vi "Incoming Signals.vi"(8 "error in (no error)":errorcluster, 11 "Node Ptr":T3 format="%.0x") -> (0 "error out":errorcluster)   [LabVIEW 2009, in "NI-XNET Custom Device.lvlib"]
uses:
  NI-XNET Custom Device.lvlib
  <vilib>/NI VeriStand/Custom Device API/Custom Device Item Ref.ctl
  Add Selected.ctl
  Add All.ctl
  <vilib>/NI VeriStand/Custom Device API/Custom Device Channel.ctl
  <vilib>/NI VeriStand/Custom Device API/Custom Device Channel Type.ctl
  <vilib>/NI VeriStand/Custom Device API/Set Item Property (Variant).vi
  <vilib>/xnet/xnet.llb/XNET String To IO Name (Frame).vi
  <vilib>/NI VeriStand/Custom Device API/Get Item Property (String).vi
  <vilib>/NI VeriStand/Custom Device API/Custom Device API.lvlib
  Program Files/National Instruments/LabVIEW 2009/resource/objmgr/xnet.rc
panel:
  in  "Add All":T1
  in  "Add Signal":T2
  in  "Header 4":cluster{"Section Name":string}={"Section Name"="Signal Specifications"}
  in  "Header 3":cluster{"Section Name":string}={"Section Name"="Signal Values"}
  in  "Header 2":cluster{"Section Name":string}={"Section Name"="Signal Settings"}
  out "Unit":string
  out "Start Bit":u32
  out "Scaling Offset":dbl
  out "Scaling Factor":dbl
  out "Number of Bits":u32
  out "Minimum Value":dbl
  out "Maximum Value":dbl
  out "Default Value":dbl
  out "Data Type":u32(ring) items=["Signed", "Unsigned", "IEEE Float"]
  out "Comment":string
  out "Byte Order":u32(ring) items=["Little Endian", "Big Endian"]
  in  "Signal Selection":i32(listbox)
  in  "Header":cluster{"Section Name":string}={"Section Name"="Signal Selection"}
  in  "Delete":bool
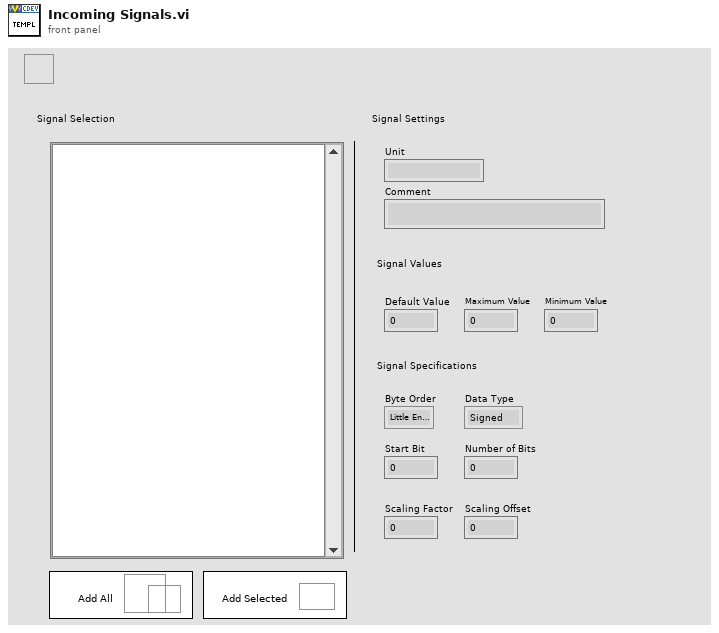
[diagram p1: front panel]
types:
  T1 = typedef "NI-XNET Custom Device.lvlib/Add All.ctl" = bool
  T2 = typedef "NI-XNET Custom Device.lvlib/Add Selected.ctl" = bool
  T3 = typedef "Custom Device API.lvlib/Custom Device Item Ref.ctl" = u64
  T4 = typedef "Custom Device API.lvlib/Custom Device Channel.ctl" = cluster{"Type":T5, "Units":string, "Default Value":dbl, "Faultable":bool, "Scalable":bool}
  T5 = typedef "Custom Device API.lvlib/Custom Device Channel Type.ctl" = enum16{"Input", "Output"}
  T6 = typedef "Custom Device API.lvlib/Custom Device Commands.ctl" = enum16{"Default", "Item renamed", "Shutdown"}
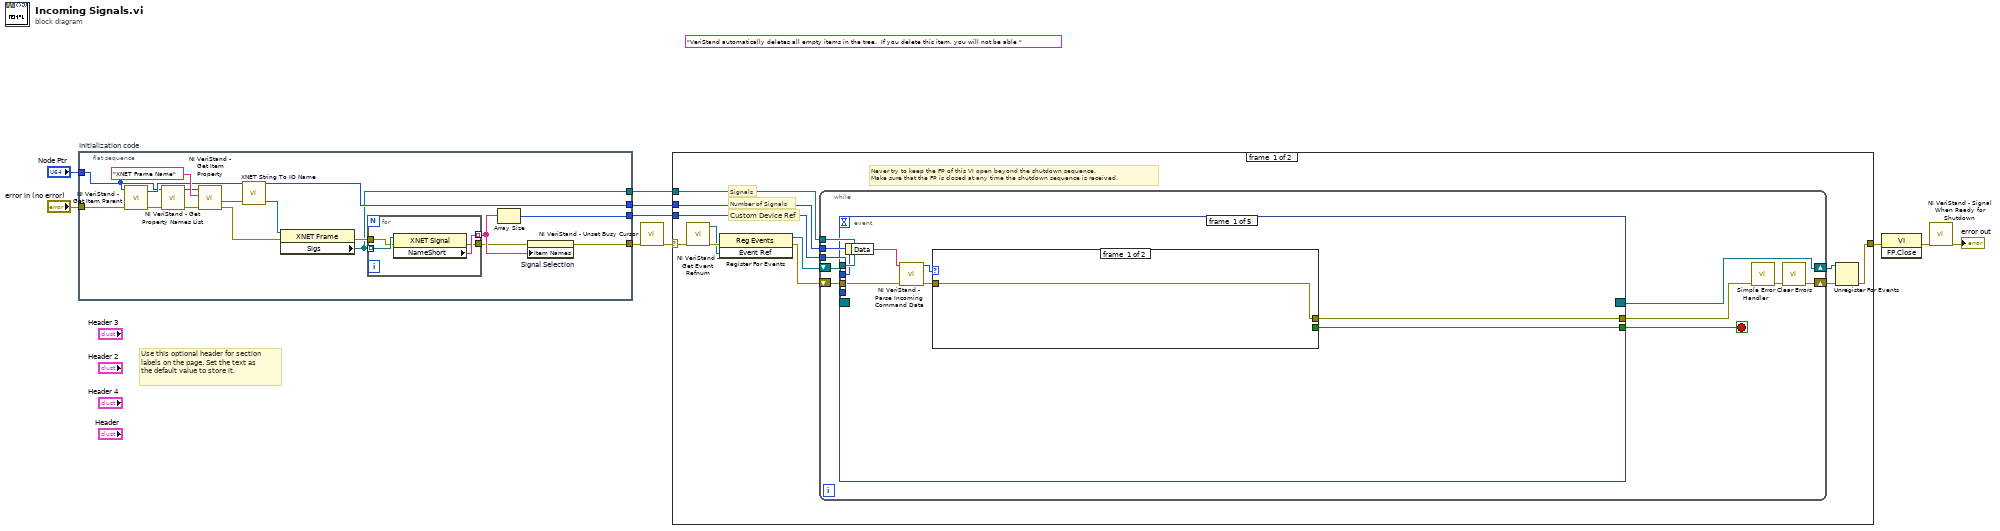
[diagram p0: block diagram]
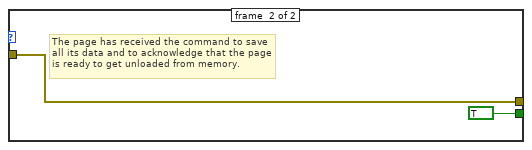
[diagram p2: hidden frame]
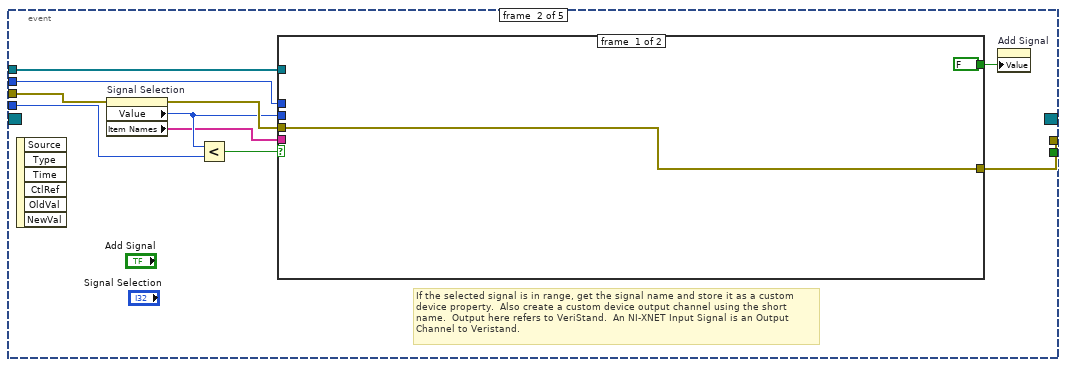
[diagram p3: hidden frame]
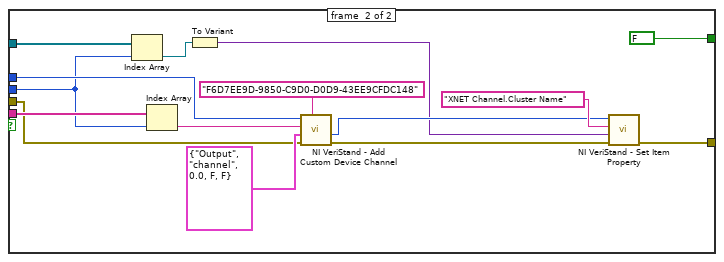
[diagram p4: hidden frame]
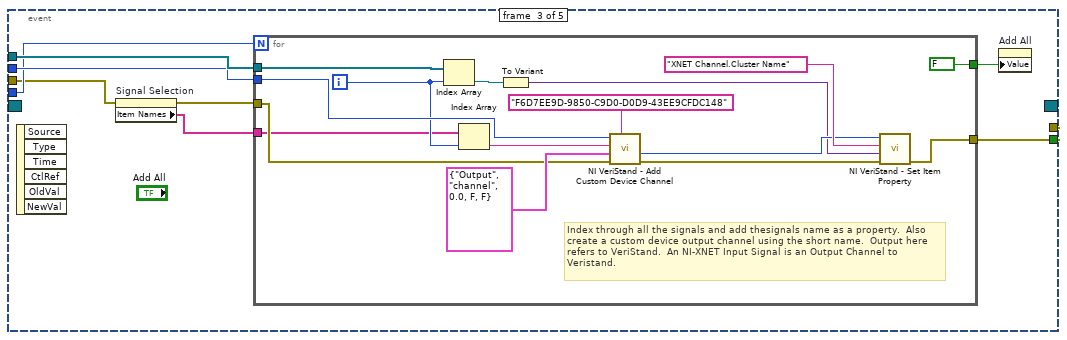
[diagram p5: hidden frame]
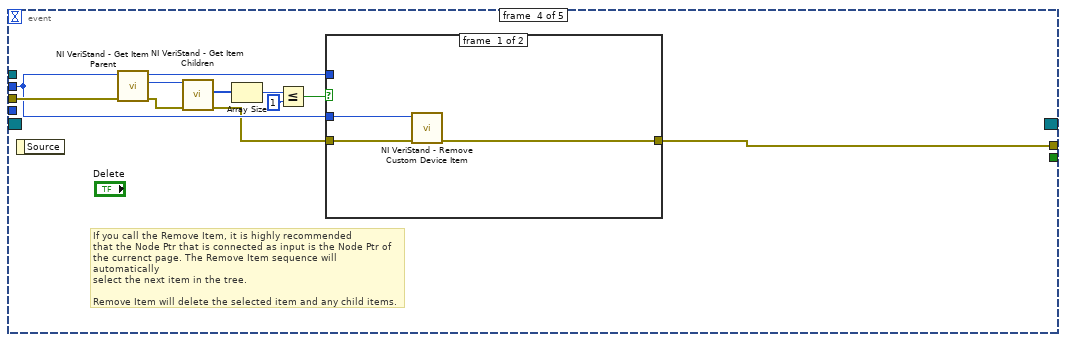
[diagram p6: hidden frame]
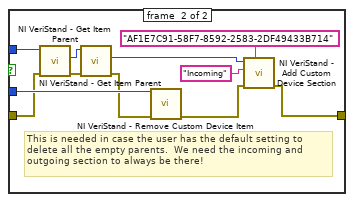
[diagram p7: hidden frame]
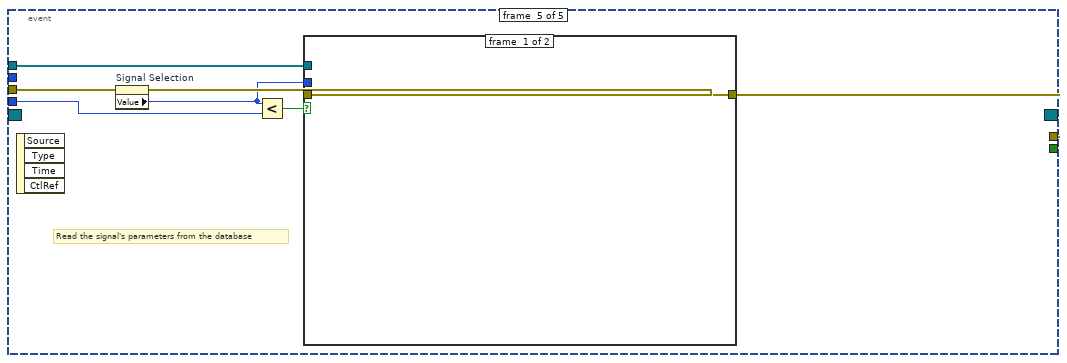
[diagram p8: hidden frame]
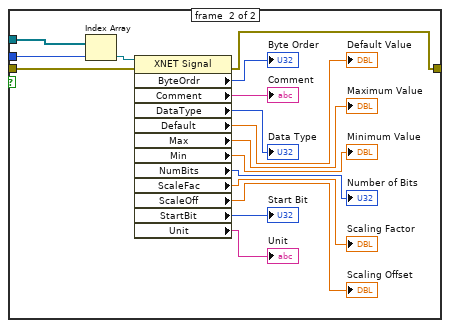
[diagram p9: hidden frame]
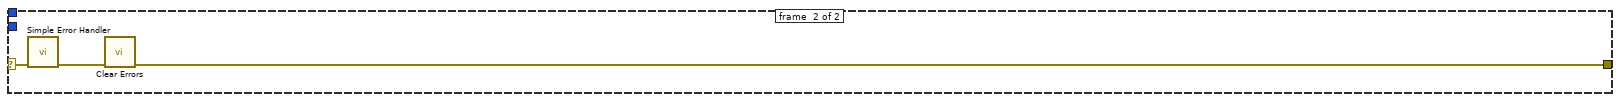
[diagram p10: hidden frame]
diagram:
  (unwired) "VeriStand automatically deletes all empty items in the tree.  If you delete this item, you will not be able " ("message")
  # "Use this optional header for section labels on the page. Set the text as the default value to store it."
  n1 = flat-sequence "Initialization code" {
    tunnel: "error in (no error)" -> [w14]
    tunnel: "Node Ptr" -> [w15]
    tunnel: [w18] -> w4
    tunnel: [w17] -> w3
    tunnel: [w16] -> w2
    tunnel: [w12] -> w1
    frame #0 {
      n2 = call <vilib>:"NI VeriStand - Get Item Parent.vi"("error in (no error)"=w14, "Parent Ref in"=w15) -> ("error out"=w25:errorcluster, "Parent Ref out"=w18:T3)  [unwired: 6 in, 2 out]
      n3 = call <vilib>:"NI VeriStand - Get Property Names List.vi"("error in (no error)"=w25, "Item Ref in"=w15) -> ("error out"=w23:errorcluster, "Item Ref out"=w24:T3)  [unwired: 7 in, 1 out]
      n4 = call-poly <vilib>:"NI VeriStand - Get Item Property.vi"("error in (no error)"=w23, "Property Name"="XNET Frame Name", "Item Ref in"=w24) -> ("error out"=w21:errorcluster, "Value"=w19:string)  [unwired: 5 in, 2 out]
      n5 = call-poly <vilib>:"XNET String To IO Name.vi"("string"=w19) -> ("XNET Frame"=w22:refnum<k21>)  [unwired: 4 in]
      n6 = property class="XNET Frame"(reference=w22, error in=w21) -> (error out=w20:errorcluster, "Sigs"=w17:refnum<k21>[])  [unwired: 1 out]
      n7 = for {
        tunnel: w17 -> [w30] mode=indexing
        tunnel: [w29] -> w13 mode=indexing
        tunnel: w20 -> [w28]
        tunnel: [w27] -> w11
        n8 = property class="XNET Signal"(reference=w30, error in=w28) -> (error out=w27:errorcluster, "NameShort"=w29:string)  [unwired: 1 out]
      }
      n9 = Array Size(array=w13) -> (size(s)=w16:i32)
      n10 = property on="Signal Selection" class="LstBox (strict)"(error in=w11, "Item Names"=w13) -> (error out=w12:errorcluster)  [unwired: 1 in, 1 out]
    }
  }
  n11 = call <vilib>:"NI VeriStand - Unset Busy Cursor.vi"("error in (no error)"=w1) -> ("error out"=w6:errorcluster)  [unwired: 10 out]
  n12 = case shown="No Error" w6 {
    selector: w6 -> [w34 w162]
    tunnel: [w38 w160] -> w10
    tunnel: w4 -> [w32 _]
    tunnel: w3 -> [w33 _]
    tunnel: w2 -> [w31 _]
    frame #0 {
      # "Custom Device Ref"
      # "Number of Signals"
      # "Signals"
      # "Never try to keep the FP of this VI open beyond the shutdown sequence.\nMake sure that the FP is closed at any time the shutdown sequence is received."
      n13 = call <vilib>:"NI VeriStand - Get Event Refnum.vi"("error in (no error)"=w34) -> ("error out"=w41:errorcluster, "Event Ref"=w37:refnum<user-event>)  [unwired: 9 out]
      n14 = register-events(error in=w41, w37) -> (reference out=w35:refnum<event-registration>, error out=w36:errorcluster)  [unwired: 1 in]
      n15 = while {
        shift-right: [w45] -> w39
        shift-left: w36 -> [w50]
        shift-right: [w51] -> w40
        shift-left: w35 -> [w49]
        tunnel: w33 -> [w44]
        tunnel: w32 -> [w43]
        tunnel: w31 -> [w42]
        stop <- w48 stop-if-true
        n16 = event shown="[3] \"Delete\": Value Change" {
          selector: w49 -> [_ _ _ _ _]
          dyn-events: [_ _ _ _ _] -> w51
          timeout: _ -> [_ _ _ _ _]
          tunnel: w50 -> [w57 w68 w89 w120 w140]
          tunnel: [w53 _ _ _ _] -> w48
          tunnel: [w52 w67 w93 w121 w141] -> w47
          tunnel: w44 -> [_ w70 w95 _ w142]
          tunnel: w43 -> [_ w69 w94 w119 _]
          tunnel: w42 -> [_ w65 w92 _ w138]
          event #0 {
            n17 = event-data() -> ("Data"=w56:string)  [unwired: 1 out]
            n18 = call <vilib>:"NI VeriStand - Parse Incoming Command Data.vi"("error in (no error)"=w57, "Data"=w56) -> ("error out"=w55:errorcluster, "Action"=w54:T6)  [unwired: 8 out]
            n19 = case shown="\"Shutdown\"" w54 {
              tunnel: w55 -> [w58 w59]
              tunnel: [_ TRUE] -> w53
              tunnel: [w58 w59] -> w52
              frame #0 {
              }
              frame #1 {
                # "The page has received the command to save all its data and to acknowledge that the page is ready to get unloaded from memory."
              }
            }
          }
          event #1 {
            # "If the selected signal is in range, get the signal name and store it as a custom device property.  Also create a custom device output channel using the short name.  Output here refers to VeriStand.  An NI-XNET Input Signal is an Output Channel to Veristand."
            n20 = event-data() -> ()  [unwired: 7 out]
            n21 = property on="Signal Selection" class="LstBox (strict)"(error in=w68) -> (error out=w66:errorcluster, "Value"=w62:i32, "Item Names"=w61:string[])  [unwired: 1 in, 1 out]
            n22 = Less?(x=w62, y=w65) -> (x < y?=w64:bool)
            n23 = case shown="True" w64 {
              tunnel: w70 -> [_ w87]
              tunnel: w69 -> [_ w86]
              tunnel: [w72 w85] -> w67
              tunnel: w61 -> [_ w78]
              tunnel: w66 -> [w72 w76]
              tunnel: w62 -> [_ w74]
              tunnel: [FALSE FALSE] -> w63
              frame #0 {
              }
              frame #1 {
                n24 = Index Array(array=w87, index=w74) -> (element=w80:refnum<k21>)
                n25 = Index Array(array=w78, index=w74) -> (element=w77:string)
                n26 = To Variant(anything=w80) -> (Variant=w79:variant)
                n27 = call <vilib>:"NI VeriStand - Add Custom Device Channel.vi"("GUID (Default Channel)"="F6D7EE9D-9850-C9D0-D0D9-43EE9CFDC148", "error in (no error)"=w76, "Channel"=T4 {"Type"=enum."Output", "Units"="channel", "Default Value"=0.0, "Faultable"=FALSE, "Scalable"=FALSE}, "Channel Name"=w77, "Parent Ref in"=w86) -> ("error out"=w75:errorcluster, "Channel Ref"=w81:T3)  [unwired: 4 in, 1 out]
                n28 = call-poly <vilib>:"NI VeriStand - Set Item Property.vi"("error in (no error)"=w75, "Value"=w79, "Property Name"="XNET Channel.Cluster Name", "Item Ref in"=w81) -> ("error out"=w85:errorcluster)  [unwired: 5 in, 2 out]
              }
            }
            n29 = property on="Add Signal" class="Bool (strict)"("Value"=w63) -> ()  [unwired: 2 in, 2 out]
          }
          event #2 {
            n30 = event-data() -> ()  [unwired: 7 out]
            n31 = property on="Signal Selection" class="LstBox (strict)"(error in=w89) -> (error out=w90:errorcluster, "Item Names"=w88:string[])  [unwired: 1 in, 1 out]
            n32 = for {
              N: w92 -> [_]
              tunnel: w95 -> [w110]
              tunnel: w94 -> [w109]
              tunnel: [w108] -> w93
              tunnel: w90 -> [w98]
              tunnel: [FALSE] -> w91
              tunnel: w88 -> [w96]
              i -> [w99]
              # "Index through all the signals and add thesignals name as a property.  Also create a custom device output channel using the short name.  Output here refers to VeriStand.  An NI-XNET Input Signal is an Output Channel to Veristand."
              n33 = Index Array(array=w110, index=w99) -> (element=w103:refnum<k21>)
              n34 = Index Array(array=w96, index=w99) -> (element=w101:string)
              n35 = To Variant(anything=w103) -> (Variant=w102:variant)
              n36 = call <vilib>:"NI VeriStand - Add Custom Device Channel.vi"("GUID (Default Channel)"="F6D7EE9D-9850-C9D0-D0D9-43EE9CFDC148", "error in (no error)"=w98, "Channel"=T4 {"Type"=enum."Output", "Units"="channel", "Default Value"=0.0, "Faultable"=FALSE, "Scalable"=FALSE}, "Channel Name"=w101, "Parent Ref in"=w109) -> ("error out"=w100:errorcluster, "Channel Ref"=w104:T3)  [unwired: 4 in, 1 out]
              n37 = call-poly <vilib>:"NI VeriStand - Set Item Property.vi"("error in (no error)"=w100, "Value"=w102, "Property Name"="XNET Channel.Cluster Name", "Item Ref in"=w104) -> ("error out"=w108:errorcluster)  [unwired: 5 in, 2 out]
            }
            n38 = property on="Add All" class="Bool (strict)"("Value"=w91) -> ()  [unwired: 2 in, 2 out]
          }
          event #3 {
            # "If you call the Remove Item, it is highly recommended\nthat the Node Ptr that is connected as input is the Node Ptr of\nthe currenct page. The Remove Item sequence will automatically\nselect the next item in the tree.\n\nRemove Item will delete the selected item and any child items."
            n39 = event-data() -> ()  [unwired: 2 out]
            n40 = call <vilib>:"NI VeriStand - Get Item Parent.vi"("error in (no error)"=w120, "Parent Ref in"=w119) -> ("error out"=w117:errorcluster, "Parent Ref"=w118:T3, "Parent Ref out"=w111:T3)  [unwired: 6 in, 1 out]
            n41 = call <vilib>:"NI VeriStand - Get Item Children.vi"("error in (no error)"=w117, "Item Ref in"=w118) -> ("error out"=w113:errorcluster, "Child Refs"=w116:T3[])  [unwired: 6 in, 2 out]
            n42 = Array Size(array=w116) -> (size(s)=w115:i32)
            n43 = Less Or Equal?(x=w115, y=1) -> (x <= y?=w112:bool)
            n44 = case shown="True" w112 {
              tunnel: [w124 w130] -> w121
              tunnel: w119 -> [w123 w132]
              tunnel: w113 -> [w122 w129]
              tunnel: w111 -> [_ w135]
              frame #0 {
                n45 = call <vilib>:"NI VeriStand - Remove Custom Device Item.vi"("error in (no error)"=w122, "Item Ref in"=w123) -> ("error out"=w124:errorcluster)  [unwired: 1 in, 8 out]
              }
              frame #1 {
                # "This is needed in case the user has the default setting to delete all the empty parents.  We need the incoming and outgoing section to always be there!"
                n46 = call <vilib>:"NI VeriStand - Get Item Parent.vi"("error in (no error)"=w129, "Parent Ref in"=w135) -> ("error out"=w127:errorcluster, "Parent Ref"=w128:T3)  [unwired: 6 in, 2 out]
                n47 = call <vilib>:"NI VeriStand - Get Item Parent.vi"("error in (no error)"=w127, "Parent Ref in"=w128) -> ("error out"=w126:errorcluster, "Parent Ref"=w125:T3)  [unwired: 6 in, 2 out]
                n48 = call <vilib>:"NI VeriStand - Remove Custom Device Item.vi"("error in (no error)"=w126, "Item Ref in"=w132) -> ("error out"=w131:errorcluster)  [unwired: 1 in, 8 out]
                n49 = call <vilib>:"NI VeriStand - Add Custom Device Section.vi"("GUID (Default Section)"="AF1E7C91-58F7-8592-2583-2DF49433B714", "error in (no error)"=w131, "Section Name"="Incoming", "Parent Ref in"=w125) -> ("error out"=w130:errorcluster)  [unwired: 5 in, 2 out]
              }
            }
          }
          event #4 {
            # "Read the signal's parameters from the database"
            n50 = event-data() -> ()  [unwired: 5 out]
            n51 = property on="Signal Selection" class="LstBox (strict)"(error in=w140) -> (error out=w139:errorcluster, "Value"=w136:i32)  [unwired: 1 in, 1 out]
            n52 = Less?(x=w136, y=w138) -> (x < y?=w137:bool)
            n53 = case shown="True" w137 {
              tunnel: w142 -> [_ w159]
              tunnel: [w143 w146] -> w141
              tunnel: w139 -> [w143 w145]
              tunnel: w136 -> [_ w144]
              frame #0 {
              }
              frame #1 {
                n54 = Index Array(array=w159, index=w144) -> (element=w158:refnum<k21>)
                n55 = property class="XNET Signal"(reference=w158, error in=w145) -> (error out=w146:errorcluster, "ByteOrdr"=→"Byte Order":u32, "Comment"=→"Comment":string, "DataType"=→"Data Type":u32, "Default"=→"Default Value":dbl, "Max"=→"Maximum Value":dbl, "Min"=→"Minimum Value":dbl, "NumBits"=→"Number of Bits":u32, "ScaleFac"=→"Scaling Factor":dbl, "ScaleOff"=→"Scaling Offset":dbl, "StartBit"=→"Start Bit":u32, "Unit"=→"Unit":string)  [unwired: 1 out]
              }
            }
          }
        }
        n56 = call <vilib>:"Simple Error Handler.vi"("error in (no error)"=w47) -> ("error out"=w46:errorcluster)  [unwired: 1 in, 7 out]
        n57 = call <vilib>:"Clear Errors.vi"("error in (no error)"=w46) -> ("error out"=w45:errorcluster)  [unwired: 6 out]
      }
      n58 = Unregister For Events(event registration refnum=w40, error in=w39) -> (error out=w38:errorcluster)
    }
    frame #1 {
      n59 = call <vilib>:"Simple Error Handler.vi"("error in (no error)"=w162) -> ("error out"=w161:errorcluster)  [unwired: 1 in, 7 out]
      n60 = call <vilib>:"Clear Errors.vi"("error in (no error)"=w161) -> ("error out"=w160:errorcluster)  [unwired: 6 out]
    }
  }
  n61 = invoke class="VI" method="FP.Close"(error in=w10) -> (error out=w9:errorcluster)  [unwired: 2 in, 2 out]
  n62 = call <vilib>:"NI VeriStand - Signal When Ready for Shutdown.vi"("error in (no error)"=w9) -> ("error out"=→"error out":errorcluster)  [unwired: 10 out]
